vi "VI_CarteNI.vi"() -> ()   [LabVIEW 2015]
uses:
  <vilib>/Utility/error.llb/DialogType.ctl
panel:
  in  "stop":bool
  in  "DIO Port 1:4-7":T1(array[cluster])=[{"Direction"=TRUE, "Drive"=FALSE, "State"=FALSE, "Pin+Name"="Pin 3, P1.7", "PhyName"="/port1/line7"}, {"Direction"=TRUE, "Drive"=FALSE, "State"=FALSE, "Pin+Name"="Pin 4, P1.6", "PhyName"="/port1/line6"}, {"Direction"=TRUE, "Drive"=FALSE, "State"=FALSE, "Pin+Name"="Pin 5, P1.5", "PhyName"="/port1/line5"}, {"Direction"=TRUE, "Drive"=FALSE, "State"=FALSE, "Pin+Name"="Pin 6, P1.4", "PhyName"="/port1/line4"}]
  in  "DIO Port 1:0-3":T1(array[cluster])=[{"Direction"=TRUE, "Drive"=FALSE, "State"=FALSE, "Pin+Name"="Pin 27, P1.0", "PhyName"="/port1/line0"}, {"Direction"=TRUE, "Drive"=FALSE, "State"=FALSE, "Pin+Name"="Pin 28, P1.1", "PhyName"="/port1/line1"}, {"Direction"=TRUE, "Drive"=FALSE, "State"=FALSE, "Pin+Name"="Pin 29, P1.2", "PhyName"="/port1/line2"}, {"Direction"=TRUE, "Drive"=FALSE, "State"=FALSE, "Pin+Name"="Pin 30, P1.3", "PhyName"="/port1/line3"}]
  in  "DIO Port 0":T1(array[cluster])=[{"Direction"=TRUE, "Drive"=FALSE, "State"=FALSE, "Pin+Name"="Pin 17, P0.0", "PhyName"="/port0/line0"}, {"Direction"=TRUE, "Drive"=FALSE, "State"=FALSE, "Pin+Name"="Pin 18, P0.1", "PhyName"="/port0/line1"}, {"Direction"=TRUE, "Drive"=FALSE, "State"=FALSE, "Pin+Name"="Pin 19, P0.2", "PhyName"="/port0/line2"}, {"Direction"=TRUE, "Drive"=FALSE, "State"=FALSE, "Pin+Name"="Pin 20, P0.3", "PhyName"="/port0/line3"}, {"Direction"=TRUE, "Drive"=FALSE, "State"=FALSE, "Pin+Name"="Pin 21, P0.4", "PhyName"="/port0/line4"}, {"Direction"=TRUE, "Drive"=FALSE, "State"=FALSE, "Pin+Name"="Pin 22, P0.5", "PhyName"="/port0/line5"}, {"Direction"=TRUE, "Drive"=FALSE, "State"=FALSE, "Pin+Name"="Pin 23, P0.6", "PhyName"="/port0/line6"}, {"Direction"=TRUE, "Drive"=FALSE, "State"=FALSE, "Pin+Name"="Pin 24, P0.7", "PhyName"="/port0/line7"}]
  out "Activity":bool=TRUE
  in  "Device Name":string="Dev1"
  in  "DIO Port 2":T1(array[cluster])=[{"Direction"=TRUE, "Drive"=FALSE, "State"=FALSE, "Pin+Name"="Pin 9, P2.7", "PhyName"="/port2/line7"}, {"Direction"=TRUE, "Drive"=FALSE, "State"=FALSE, "Pin+Name"="Pin 10, P2.6", "PhyName"="/port2/line6"}, {"Direction"=TRUE, "Drive"=FALSE, "State"=FALSE, "Pin+Name"="Pin 11, P2.5", "PhyName"="/port2/line5"}, {"Direction"=TRUE, "Drive"=FALSE, "State"=FALSE, "Pin+Name"="Pin 12, P2.4", "PhyName"="/port2/line4"}, {"Direction"=TRUE, "Drive"=FALSE, "State"=FALSE, "Pin+Name"="Pin 13, P2.3", "PhyName"="/port2/line3"}, {"Direction"=TRUE, "Drive"=FALSE, "State"=FALSE, "Pin+Name"="Pin14, P2.2", "PhyName"="/port2/line2"}, {"Direction"=TRUE, "Drive"=FALSE, "State"=FALSE, "Pin+Name"="Pin 15, P2.1", "PhyName"="/port2/line1"}, {"Direction"=TRUE, "Drive"=FALSE, "State"=FALSE, "Pin+Name"="Pin 16, P2.0", "PhyName"="/port2/line0"}]
  # "Entrée/Sortie"
  # "Etat"
  # "Entrée/Sortie"
  # "Etat"
  # "Vérin bridage sorti"
  # "Départ cycle"
  # "Vérin marquage sorti"
  # "Présence air"
  # "Posage"
  # "Sécurité porte 2"
  # "Sécurité porte 1"
  # "Sens antihorraire Moteur2"
  # "Entrer Vérin porte"
  # "Sens horraire Moteur2"
  # "Sortir Vérin marquage"
  # "Sens antihorraire Moteur1"
  # "Sortir Vérin bridage"
  # "Sens horraire Moteur1"
  # "Eclairage Led"
  # "Sortir Vérin porte"
  # "Vérin Porte sorti"
  # "Entrer Vérin Chariot"
  # "Vérin Porte entré"
  # "Sortir Vérin Chariot"
  # "Vérin Chariot sorti"
  # "Activer Terminal 1"
  # "Vérin chariot entré"
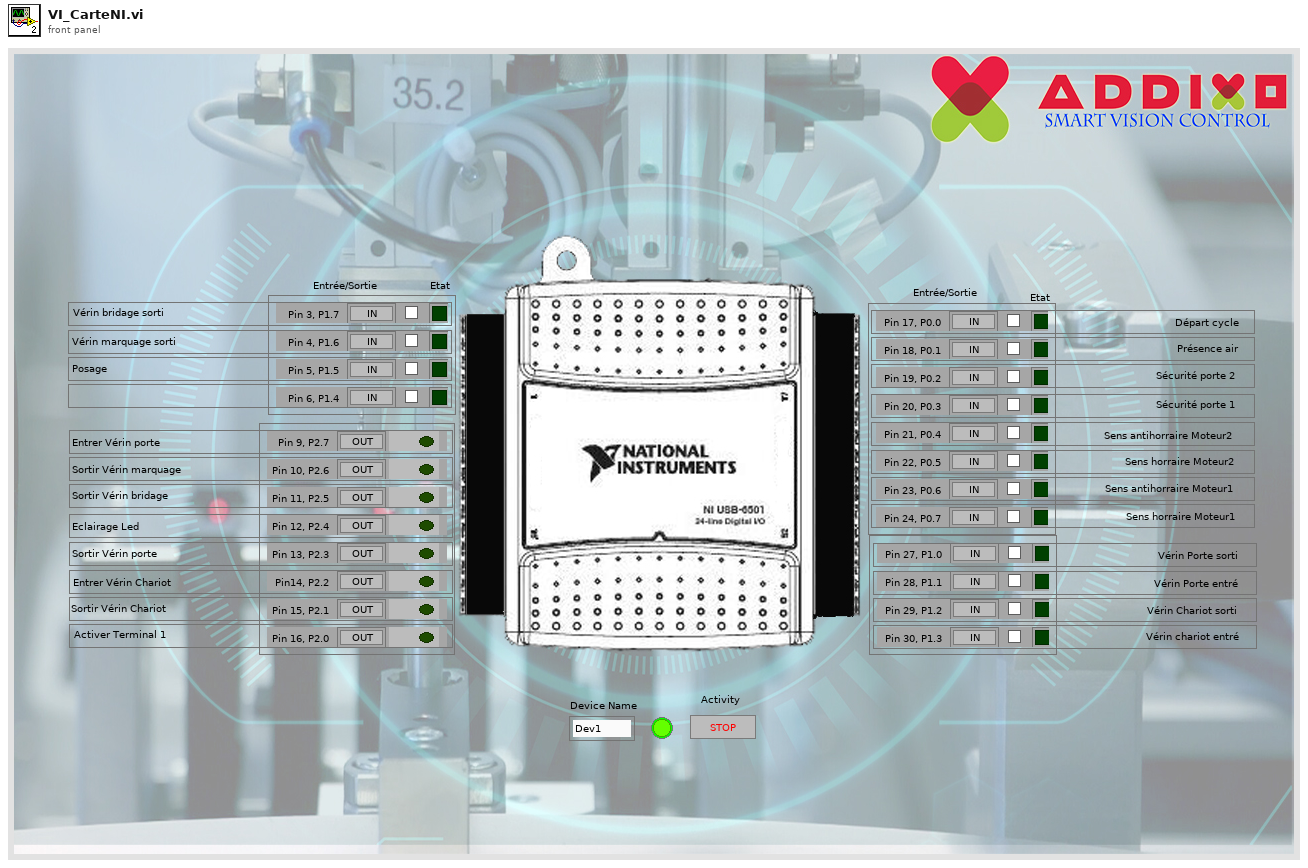
[diagram p1: front panel]
types:
  T1 = cluster{"Direction":bool, "Drive":bool, "State":bool, "Pin+Name":string, "PhyName":string}[]
  T2 = typedef "DialogType.ctl" = u16
  T3 = cluster{"Direction":bool, "Drive":bool, "State":bool, "Pin+Name":string, "PhyName":string}
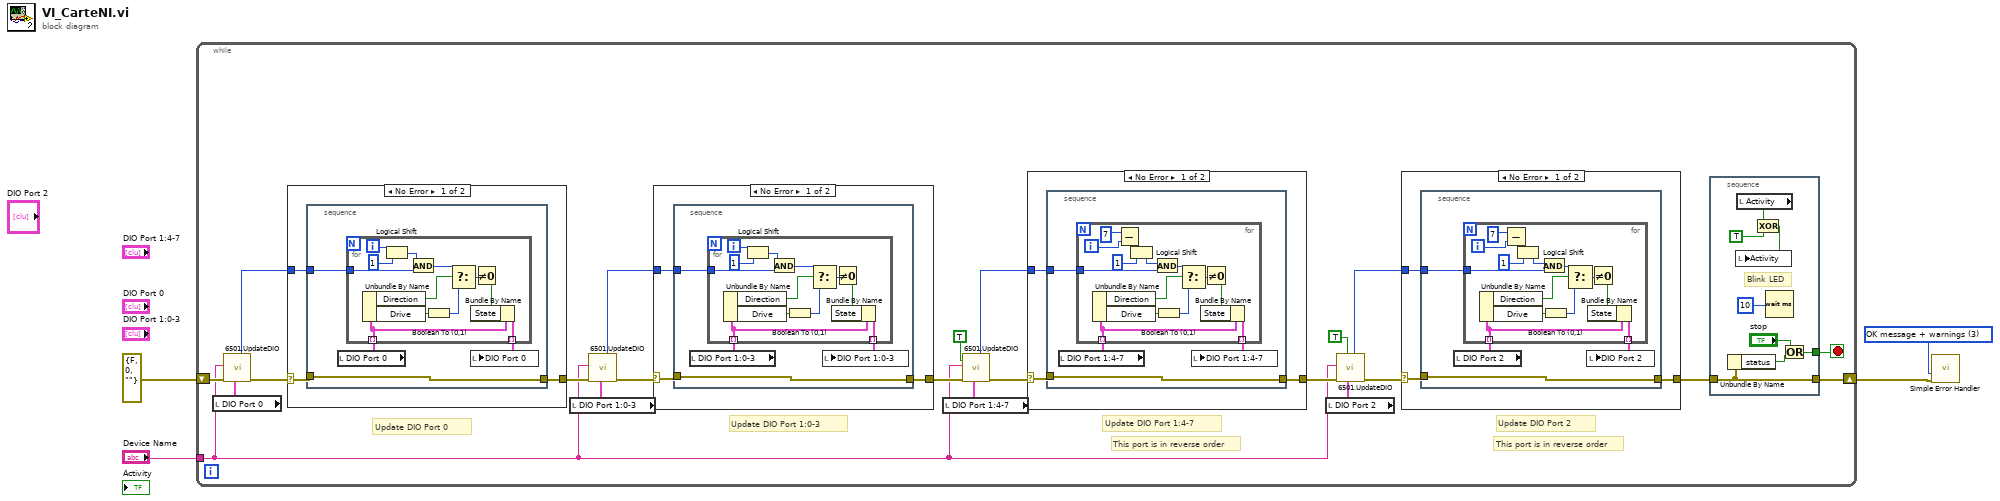
[diagram p0: block diagram]
diagram:
  w4 = T2 3 items=["no dialog", "OK message", "continue or stop message", "OK message + warnings", "continue/stop + warnings"] ("type of dialog (OK msg:1)")
  n1 = while {
    shift-right: [w19] -> w3
    shift-left: errorcluster {"status"=FALSE, "code"=0, "source"=""} ("error IO") -> [w17]
    tunnel: "Device Name" -> [w7]
    stop <- w18 stop-if-true
    # "This port is in reverse order"
    # "Update DIO Port 2"
    # "This port is in reverse order"
    # "Update DIO Port 1:4-7"
    # "Update DIO Port 1:0-3"
    # "Update DIO Port 0"
    n2 = local read "DIO Port 0"() -> (w25:T1)
    n3 = call "6501.UpdateDIO.vi"("DIO Port"=w25, "error in"=w17, "Device Name"=w7) -> ("error out"=w20:errorcluster, "Port Value"=w26:i32)  [unwired: 7 in]
    n4 = case shown="No Error" w20 {
      selector: w20 -> [w79 w98]
      tunnel: w26 -> [w81 _]
      tunnel: [w80 w98] -> w24
      frame No Error {
        n5 = stacked-sequence {
          tunnel: w79 -> [w85]
          tunnel: [w85] -> w80
          tunnel: w81 -> [w82]
          frame #0 {
            n6 = local read "DIO Port 0"() -> (w84:T1)
            n7 = for {
              tunnel: w82 -> [w89]
              tunnel: w84 -> [w86] mode=indexing
              tunnel: [w87] -> w83 mode=indexing
              i -> [w95]
              n8 = Unbundle By Name(w86) -> ("Direction"=w88:bool, "Drive"=w90:bool)
              n9 = Logical Shift(y=w95, x=1) -> (x << y=w93:i32)
              n10 = And(x=w93, y=w89) -> (x .and. y?=w92:i32)
              n11 = Boolean To (0,1)(Boolean=w90) -> (0, 1=w97:i16)
              n12 = Select(t=w92, s=w88, f=w97) -> (s? t:f=w96:i32)
              n13 = Not Equal To 0?(x=w96) -> (x != 0?=w91:bool)
              n14 = Bundle By Name(cluster=w86, "State"=w91) -> (w87:T3)
            }
            n15 = local write "DIO Port 0"(w83) -> ()
          }
        }
      }
      frame Error {
      }
    }
    n16 = local read "DIO Port 1:0-3"() -> (w22:T1)
    n17 = call "6501.UpdateDIO.vi"("DIO Port"=w22, "error in"=w24, "Device Name"=w7) -> ("error out"=w21:errorcluster, "Port Value"=w23:i32)  [unwired: 7 in]
    n18 = case shown="No Error" w21 {
      selector: w21 -> [w99 w118]
      tunnel: w23 -> [w101 _]
      tunnel: [w100 w118] -> w13
      frame No Error {
        n19 = stacked-sequence {
          tunnel: w99 -> [w105]
          tunnel: [w105] -> w100
          tunnel: w101 -> [w102]
          frame #0 {
            n20 = local read "DIO Port 1:0-3"() -> (w104:T1)
            n21 = for {
              tunnel: w102 -> [w109]
              tunnel: w104 -> [w106] mode=indexing
              tunnel: [w107] -> w103 mode=indexing
              i -> [w115]
              n22 = Unbundle By Name(w106) -> ("Direction"=w108:bool, "Drive"=w110:bool)
              n23 = Logical Shift(y=w115, x=1) -> (x << y=w113:i32)
              n24 = And(x=w113, y=w109) -> (x .and. y?=w112:i32)
              n25 = Boolean To (0,1)(Boolean=w110) -> (0, 1=w117:i16)
              n26 = Select(t=w112, s=w108, f=w117) -> (s? t:f=w116:i32)
              n27 = Not Equal To 0?(x=w116) -> (x != 0?=w111:bool)
              n28 = Bundle By Name(cluster=w106, "State"=w111) -> (w107:T3)
            }
            n29 = local write "DIO Port 1:0-3"(w103) -> ()
          }
        }
      }
      frame Error {
      }
    }
    n30 = local read "DIO Port 1:4-7"() -> (w15:T1)
    n31 = call "6501.UpdateDIO.vi"("DIO Port"=w15, "Reverse"=TRUE, "error in"=w13, "Device Name"=w7) -> ("error out"=w16:errorcluster, "Port Value"=w14:i32)  [unwired: 6 in]
    n32 = case shown="No Error" w16 {
      selector: w16 -> [w49 w70]
      tunnel: w14 -> [w51 _]
      tunnel: [w50 w70] -> w10
      frame No Error {
        n33 = stacked-sequence {
          tunnel: w49 -> [w55]
          tunnel: [w55] -> w50
          tunnel: w51 -> [w52]
          frame #0 {
            n34 = local read "DIO Port 1:4-7"() -> (w54:T1)
            n35 = for {
              tunnel: w52 -> [w62]
              tunnel: w54 -> [w59] mode=indexing
              tunnel: [w60] -> w53 mode=indexing
              i -> [w57]
              n36 = Unbundle By Name(w59) -> ("Direction"=w61:bool, "Drive"=w63:bool)
              n37 = Subtract(x=7, y=w57) -> (x-y=w56:i32)
              n38 = Logical Shift(y=w56, x=1) -> (x << y=w66:i32)
              n39 = And(x=w66, y=w62) -> (x .and. y?=w65:i32)
              n40 = Boolean To (0,1)(Boolean=w63) -> (0, 1=w69:i16)
              n41 = Select(t=w65, s=w61, f=w69) -> (s? t:f=w68:i32)
              n42 = Not Equal To 0?(x=w68) -> (x != 0?=w64:bool)
              n43 = Bundle By Name(cluster=w59, "State"=w64) -> (w60:T3)
            }
            n44 = local write "DIO Port 1:4-7"(w53) -> ()
          }
        }
      }
      frame Error {
      }
    }
    n45 = local read "DIO Port 2"() -> (w11:T1)
    n46 = call "6501.UpdateDIO.vi"("DIO Port"=w11, "Reverse"=TRUE, "error in"=w10, "Device Name"=w7) -> ("error out"=w9:errorcluster, "Port Value"=w12:i32)  [unwired: 6 in]
    n47 = case shown="No Error" w9 {
      selector: w9 -> [w27 w48]
      tunnel: w12 -> [w29 _]
      tunnel: [w28 w48] -> w8
      frame No Error {
        n48 = stacked-sequence {
          tunnel: w27 -> [w33]
          tunnel: [w33] -> w28
          tunnel: w29 -> [w30]
          frame #0 {
            n49 = local read "DIO Port 2"() -> (w32:T1)
            n50 = for {
              tunnel: w30 -> [w40]
              tunnel: w32 -> [w37] mode=indexing
              tunnel: [w38] -> w31 mode=indexing
              i -> [w35]
              n51 = Unbundle By Name(w37) -> ("Direction"=w39:bool, "Drive"=w41:bool)
              n52 = Subtract(x=7, y=w35) -> (x-y=w34:i32)
              n53 = Logical Shift(y=w34, x=1) -> (x << y=w44:i32)
              n54 = And(x=w44, y=w40) -> (x .and. y?=w43:i32)
              n55 = Boolean To (0,1)(Boolean=w41) -> (0, 1=w47:i16)
              n56 = Select(t=w43, s=w39, f=w47) -> (s? t:f=w46:i32)
              n57 = Not Equal To 0?(x=w46) -> (x != 0?=w42:bool)
              n58 = Bundle By Name(cluster=w37, "State"=w42) -> (w38:T3)
            }
            n59 = local write "DIO Port 2"(w31) -> ()
          }
        }
      }
      frame Error {
      }
    }
    n60 = stacked-sequence {
      tunnel: w8 -> [w71]
      tunnel: [w76] -> w18
      tunnel: [w71] -> w19
      frame #0 {
        # "Blink LED"
        n61 = Unbundle By Name(w71) -> ("status"=w78:bool)
        n62 = local read "Activity"() -> (w73:bool)
        n63 = Exclusive Or(1:TRUE, 2:w73) -> (0:w75:bool)
        n64 = local write "Activity"(w75) -> ()
        n65 = Wait (ms)(milliseconds to wait=10) -> ()  [unwired: 1 out]
        n66 = Or(x="stop", y=w78) -> (x .or. y?=w76:bool)
      }
    }
  }
  n67 = call <vilib>:"Simple Error Handler.vi"("type of dialog (OK msg:1)"=w4, "error in (no error)"=w3) -> ()  [unwired: 3 in, 5 out]
